vi "CCC Stop Server.vi"(8 "error in (no error)":errorcluster, 9 "timeout ms (1000)":i32=1000, 10 "abort (F)":bool) -> (0 "error out":errorcluster)   [LabVIEW 2010]
doc: "Stops the CCC server process."
uses:
  NI_CCC.lvlib
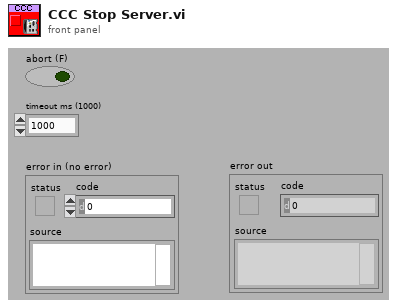
[diagram p1: front panel]
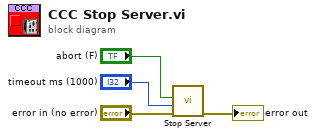
[diagram p0: block diagram]
diagram:
  n1 = call "Stop Server.vi"("error in"="error in (no error)", "timeout ms (1000)"="timeout ms (1000)", "abort (F)"="abort (F)") -> ("error out"=→"error out":errorcluster)  [unwired: 8 in]
